vi "Post-Project-Copying Process - Stage 3.vi"(8 "error in":errorcluster, 11 "PluginGenerator_MetaDataObj":refnum<class "PluginGenerator_MetaDataObj.lvclass">) -> (0 "error out":errorcluster, 3 "PluginGenerator_MetaDataObj out":refnum<class "PluginGenerator_MetaDataObj.lvclass">)   [LabVIEW 2021, in "Plugin Generator.lvlib"]
uses:
  Plugin Generator.lvlib
  <vilib>/Utility/EditLVProj/Edit LVProj.lvlib
  PluginGenerator_MetaDataObj/PluginGenerator_MetaDataObj.lvclass
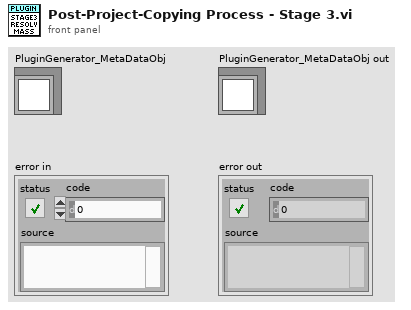
[diagram p1: front panel]
types:
  T1 = typedef "Plugin Generator.lvlib/Plugin OS.ctl" = enum16{"Linux RT", "Env Server"}
  T2 = typedef "Edit LVProj.lvlib/Library And VI References.ctl" = cluster{"Target Reference":refnum<vi>, "VI References":refnum<vi>[], "Library References":refnum<vi>[]}
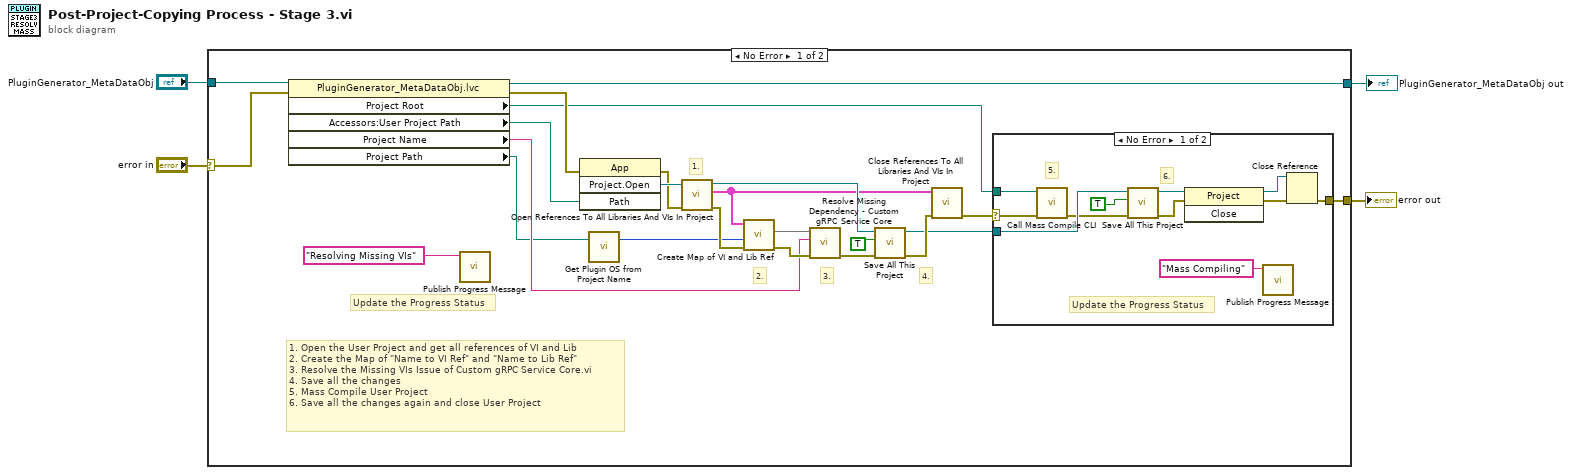
[diagram p0: block diagram]
diagram:
  n1 = case shown="No Error" "error in" {
    selector: "error in" -> [w9 w41]
    tunnel: [w27 w41] -> w4
    tunnel: "PluginGenerator_MetaDataObj" -> [w26 w40]
    tunnel: [w25 w40] -> w2
    frame No Error {
      # "4."
      # "3."
      # "2."
      # "1. Open the User Project and get all references of VI and Lib\n2. Create the Map of \"Name to VI Ref\" and \"Name to Lib Ref\"\n3. Resolve the Missing VIs Issue of Custom gRPC Service Core.vi\n4. Save all the changes\n5. Mass Compile User Project\n6. Save all the changes again and close User Project"
      # "1."
      # "Update the Progress Status"
      n2 = property class="PluginGenerator_MetaDataObj.lvc"(reference=w26, error in=w9) -> (reference out=w25:refnum<class "PluginGenerator_MetaDataObj.lvclass">, error out=w11:errorcluster, "Project Root"=w8:path, "Accessors:User Project Path"=w12:path, "Project Name"=w13:string, "Project Path"=w5:path)
      n3 = call "Publish Progress Message.vi"("Progress"="Resolving Missing VIs") -> ()  [unwired: 11 in]
      n4 = invoke class="App" method="Project.Open"(error in=w11, "Path"=w12) -> (error out=w23:errorcluster, "Project:Open"=w24:refnum<vi>)  [unwired: 2 in, 2 out]
      n5 = call "Get Plugin OS from Project Name.vi"("Project Path"=w5) -> ("Plugin OS"=w6:T1)  [unwired: 2 in]
      n6 = call <vilib>:"Open References To All Libraries And VIs In Project.vi"("error in (no error)"=w23, "Project in"=w24) -> ("error out"=w14:errorcluster, "VI and Library References"=w17:T2[], "Project out"=w19:refnum<vi>)  [unwired: 7 in]
      n7 = call "Create Map of VI and Lib Ref.vi"("error in"=w14, "Plugin OS"=w6, "VI and Library References"=w17) -> ("error out"=w15:errorcluster, "Map - LibRef"=w22:map{string, refnum<vi>})  [unwired: 6 in, 1 out]
      n8 = call "Resolve Missing Dependency - Custom gRPC Service Core.vi"("error in"=w15, "Project Name"=w13, "Map - LibRef"=w22) -> ("error out"=w20:errorcluster)  [unwired: 8 in]
      n9 = call <vilib>:"Save All This Project.vi"("error in (no error)"=w20, "Exclude Dependencies? (F)"=TRUE, "Project in"=w19) -> ("error out"=w18:errorcluster, "Project out"=w16:refnum<vi>)  [unwired: 7 in]
      n10 = call <vilib>:"Close References To All Libraries And VIs In Project.vi"("error in (no error)"=w18, "VI and Library References"=w17) -> ("error out"=w7:errorcluster)  [unwired: 9 in]
      n11 = case shown="No Error" w7 {
        selector: w7 -> [w28 w39]
        tunnel: [w38 w39] -> w27
        tunnel: w16 -> [w34 _]
        tunnel: w8 -> [w29 _]
        frame No Error {
          # "6."
          # "5."
          # "Update the Progress Status"
          n12 = call "Call Mass Compile CLI.vi"("error in"=w28, "Project Root"=w29) -> ("error out"=w31:errorcluster)  [unwired: 9 in]
          n13 = call <vilib>:"Save All This Project.vi"("error in (no error)"=w31, "Exclude Dependencies? (F)"=TRUE, "Project in"=w34) -> ("error out"=w35:errorcluster, "Project out"=w36:refnum<vi>)  [unwired: 7 in]
          n14 = invoke class="Project" method="Close"(reference=w36, error in=w35) -> (reference out=w33:refnum<vi>, error out=w32:errorcluster)  [unwired: 1 in, 1 out]
          n15 = call "Publish Progress Message.vi"("Progress"="Mass Compiling") -> ()  [unwired: 11 in]
          n16 = Close Reference(reference=w33, error in (no error)=w32) -> (error out=w38:errorcluster)
        }
        frame Error {
        }
      }
    }
    frame Error {
    }
  }
  "error out" <- w4
  "PluginGenerator_MetaDataObj out" <- w2
